vi "Create.vi"(6 "Buffer Size (20)":i32=20, 8 "error in (no error)":errorcluster, 10 "Settings":T1, 11 "NetworkConnection in":refnum<class "NetworkConnection.lvclass">) -> (0 "error out":errorcluster, 3 "NetworkConnection out":refnum<class "NetworkConnection.lvclass">)   [LabVIEW 2023, in "NetworkConnection.lvclass"]
doc: "Configures the instance of the Network Connection based on the provided settings. \n- My Name: Name of the connection on the local computer.\n- Remote IP: IP address of the remote system to which the connection will be made (ONLY ONE OF THE ENDPOINTS NEEDS TO SPECIFY AN IP ADDRESS).\n- Remote Name: name of the connection in the remote system to which the connection will be made.\nJKI Network Streams Connection 1.1.1.15\nJavier Ruiz - JKI\nCopyright (c) 2020, JKI\n\nThis library is provided \"AS IS\" ,WITHOUT WARRANTIES OR CONDITIONS OF ANY KIND, either express or implied."
uses:
  NetworkConnection.lvclass
  PublicSettings.ctl
  NetworkMessage.ctl
  NetworkCommand.ctl
  NetworkConnection.lvclass/NetworkConnection.ctl
panel:
  # "Copyright © 2020 JKI All rights reserved.\n\nAuthor: Javier Ruiz <javier.ruiz@jki.net>\n\nThis library is provided \"AS IS\" ,WITHOUT WARRANTIES OR \nCONDITIONS OF ANY KIND, either expressed or implied.\n\nJKI -- jki.net"
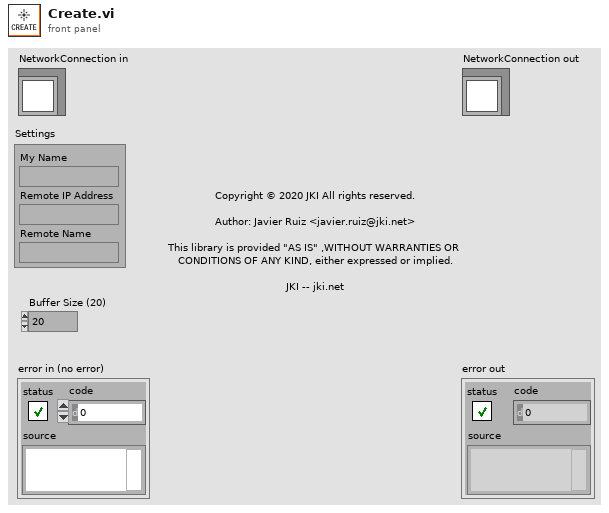
[diagram p1: front panel]
types:
  T1 = typedef "NetworkConnection.lvclass/PublicSettings.ctl" = cluster{"My Name":string, "Remote IP Address":string, "Remote Name":string}
  T2 = typedef "NetworkConnection.lvclass/NetworkMessage.ctl" = cluster{"NetworkCommand":T3, "Wait for Ack?":bool, "Ack Id":i32}
  T3 = typedef "NetworkConnection.lvclass/NetworkCommand.ctl" = cluster{"Command":string, "Arguments":variant}
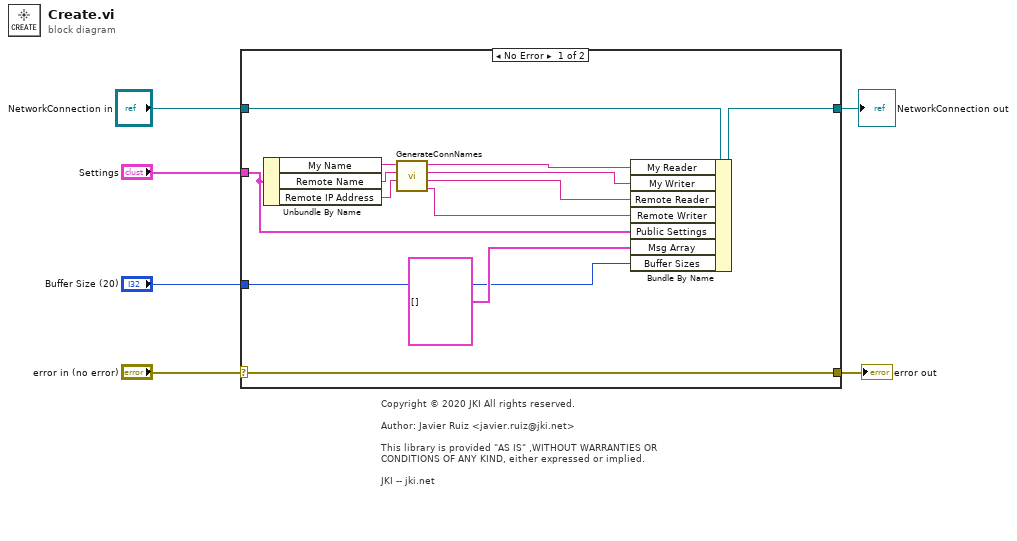
[diagram p0: block diagram]
diagram:
  # "Copyright © 2020 JKI All rights reserved.\n\nAuthor: Javier Ruiz <javier.ruiz@jki.net>\n\nThis library is provided \"AS IS\" ,WITHOUT WARRANTIES OR \nCONDITIONS OF ANY KIND, either expressed or implied.\n\nJKI -- jki.net"
  n1 = case shown="No Error" "error in (no error)" {
    selector: "error in (no error)" -> [w9 w21]
    tunnel: [w9 w21] -> w5
    tunnel: [w18 w20] -> w3
    tunnel: "NetworkConnection in" -> [w19 w20]
    tunnel: "Settings" -> [w17 _]
    tunnel: "Buffer Size (20)" -> [w8 _]
    frame No Error {
      n2 = Unbundle By Name(w17) -> ("My Name"=w11:string, "Remote Name"=w16:string, "Remote IP Address"=w7:string)
      n3 = call "GenerateConnNames.vi"("Remote IP Add"=w7, "Remote Name"=w16, "My Name"=w11) -> ("Remote Writer"=w14:string, "Remote Reader"=w12:string, "My Writer"=w13:string, "My Reader"=w15:string)  [unwired: 5 in]
      n4 = Bundle By Name(cluster=w19, "My Reader"=w15, "My Writer"=w13, "Remote Reader"=w12, "Remote Writer"=w14, "Public Settings"=w17, "Msg Array"=T2[] [], "Buffer Sizes"=w8) -> (w18:refnum<class "NetworkConnection.lvclass">)
    }
    frame Error {
    }
  }
  "error out" <- w5
  "NetworkConnection out" <- w3
